vi "SerialMarvinMod.vi"(8 "error in (no error)":errorcluster, 9 "Clear Log":bool, 10 "write buffer":string="UA[3]\r\n", 11 "VISA resource name":refnum<visa-resource-name>="COM6") -> (0 "error out":errorcluster, 2 "read buffer":string)   [LabVIEW 2017]
uses:
  <vilib>/Instr/_visa.llb/VISA Configure Serial Port (Instr).vi
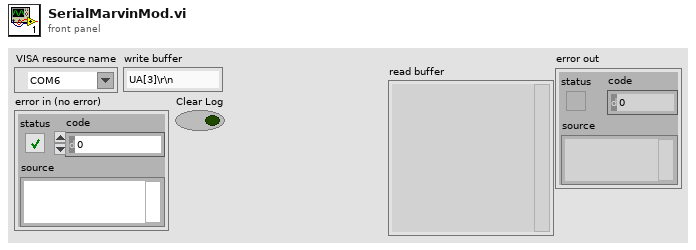
[diagram p1: front panel]
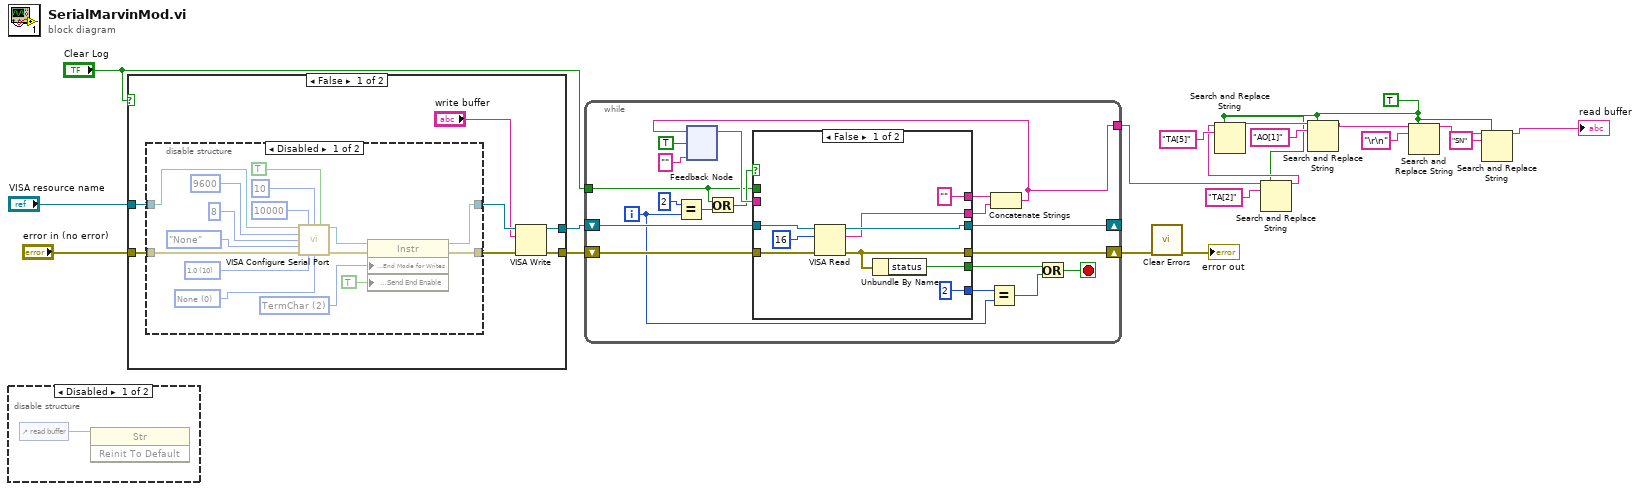
[diagram p0: block diagram]
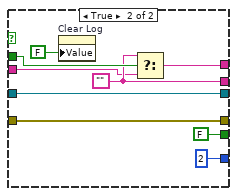
[diagram p5: hidden frame]
diagram:
  w1 = TRUE ("replace all? (F)")
  n1 = disable-structure shown="Disabled" {
    frame Disabled {
      n2 = control-ref of="read buffer"() -> (w20:refnum<vi>)
      n3 = invoke class="Str" method="Reinit To Default"(reference=w20) -> ()  [unwired: 2 in, 3 out]
    }
    frame Enabled {
    }
  }
  n4 = case shown="False" "Clear Log" {
    tunnel: "VISA resource name" -> [w27 w47]
    tunnel: "error in (no error)" -> [w26 w46]
    tunnel: [w23 w47] -> w15
    tunnel: [w22 w46] -> w14
    frame False {
      n5 = disable-structure shown="Disabled" {
        disable-tunnel: w27 -> [w43 w45]
        disable-tunnel: w26 -> [w37 w44]
        disable-tunnel: [w32 w45] -> w24
        disable-tunnel: [w31 w44] -> w25
        frame Disabled {
          w29 = u16 2 items=["None", "LastBit", "TermChar", "Break"] ("Serial Settings:Serial End Mode for Writes")
          w35 = u16 0 items=["None", "XON/XOFF", "RTS/CTS", "XON/XOFF & RTS/CTS", "DTR/DSR", "XON/XOFF & DTR/DSR"] ("flow control (0:none)")
          w36 = u16 10 items=["1.0"=10, "1.5"=15, "2.0"=20] ("stop bits (10: 1 bit)")
          n6 = call-poly "VISA Configure Serial Port"("VISA resource name"=w43, "timeout (10sec)"=u32 10000, "termination char\n(0xA = '\\n' = LF)"=u8 10 ("termination char\n(0xA = '\\n' = LF)"), "Enable Termination\nChar (T)"=TRUE ("Enable Termination\nChar (T)"), "baud rate (9600)"=u32 9600, "data bits (8)"=u16 8, "parity (0:none)"=enum16{"None", "Odd", "Even", "Mark", "Space"}."None", "error in (no error)"=w37, "stop bits (10: 1 bit)"=w36, "flow control (0:none)"=w35) -> ("VISA resource name out"=w33:refnum<visa-resource-name>, "error out"=w34:errorcluster)  [unwired: 4 in]
          n7 = property class="Instr"(reference=w33, error in=w34, "Serial Settings:End Mode for Writes"=w29, "Message Based Settings:Send End Enable"=TRUE) -> (reference out=w32:refnum<visa-resource-name>, error out=w31:errorcluster)
        }
        frame Enabled {
        }
      }
      n8 = VISA Write(VISA resource name=w24, write buffer="write buffer", error in (no error)=w25) -> (VISA resource name out=w23:refnum<visa-resource-name>, error out=w22:errorcluster)  [unwired: 1 out]
    }
    frame True {
    }
  }
  n9 = while {
    shift-right: [w66] -> _
    shift-left: w15 -> [w62]
    shift-right: [w64] -> w18
    shift-left: w14 -> [w61]
    tunnel: [w48] -> w3
    tunnel: "Clear Log" -> [w53]
    i -> [w57]
    stop <- w49 stop-if-true
    n10 = Equal?(x=2, y=w57) -> (x = y?=w55:bool)
    n11 = feedback #1("") -> (w60:string)
    n12 = Or(x=w53, y=w55) -> (x .or. y?=w54:bool)
    n13 = case shown="False" w54 {
      tunnel: [w75 w84] -> w66
      tunnel: [w74 w78] -> w65
      tunnel: [w72 w83] -> w64
      tunnel: [w71 FALSE ("status")] -> w63
      tunnel: w62 -> [w70 w84]
      tunnel: w61 -> [w69 w83]
      tunnel: w60 -> [_ w77]
      tunnel: ["" w76] -> w59
      tunnel: [2 ("x") 2 ("x")] -> w58
      tunnel: w53 -> [_ w79]
      frame False {
        n14 = VISA Read(VISA resource name=w70, byte count=u32 16, error in (no error)=w69) -> (VISA resource name out=w75:refnum<visa-resource-name>, read buffer=w74:string, error out=w72:errorcluster)  [unwired: 1 out]
        n15 = Unbundle By Name(w72) -> ("status"=w71:bool)
      }
      frame True {
        w78 = ""
        n16 = property on="Clear Log" class="Bool (strict)"("Value"=FALSE ("Clear Log")) -> ()  [unwired: 2 in, 2 out]
        n17 = Select(t=w78, s=w79, f=w77) -> (s? t:f=w76:string)
      }
    }
    n18 = Equal?(x=w58, y=w57) -> (x = y?=w50:bool)
    n19 = Concatenate Strings(w59, w65) -> (w48:string)
    n20 = feedback-in #1(w48, TRUE) -> ()
    n21 = Or(x=w63, y=w50) -> (x .or. y?=w49:bool)
  }
  n22 = call <vilib>:"Clear Errors.vi"("error in (no error)"=w18) -> ("error out"=→"error out":errorcluster)  [unwired: 5 in, 1 out]
  n23 = Search and Replace String(replace all?=w1, input string=w3, search string="TA[2]" ("substring (\"\")")) -> (result string=w2:string)  [unwired: 5 in, 3 out]
  n24 = Search and Replace String(replace all?=w1, input string=w2, search string="TA[5]" ("substring (\"\")")) -> (result string=w10:string)  [unwired: 5 in, 3 out]
  n25 = Search and Replace String(replace all?=w1, input string=w10, search string="AO[1]" ("substring (\"\")")) -> (result string=w8:string)  [unwired: 5 in, 3 out]
  n26 = Search and Replace String(replace all?=w1, input string=w8, search string="\r\n" ("substring (\"\")")) -> (result string=w7:string)  [unwired: 5 in, 3 out]
  n27 = Search and Replace String(replace all?=w1, input string=w7, search string="SN") -> (result string=→"read buffer":string)  [unwired: 5 in, 3 out]
